vi "Add Namer with Shared Approval File.vi"   [LabVIEW 2020, in "Approval Tests.lvlib"]
doc: "Drops everything needed to have several approval tests share the same approval file."
uses:
  Approval Tests.lvlib
  Options/Options.lvclass
  Namer With Shared Approved File/Namer With Shared Approved File.lvclass
  Namer With Shared Approved File/Namer With Shared Approved File.lvclass/Namer With Shared Approved File.ctl
  Namer With Shared Approved File/Write Shared Approved File Path.vi
  Options/Write Namer.vi
  C:/Users/SAS/Desktop/ApprovalTests.LabVIEW/Source/Approval Tests/Namer/Namer.lvclass
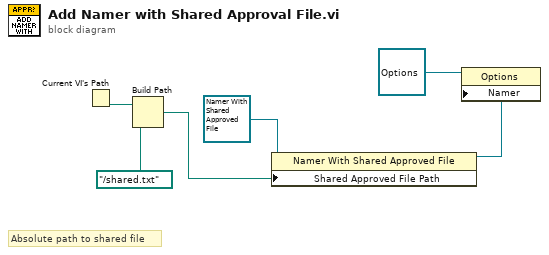
[diagram p0: block diagram]
diagram:
  # "Absolute path to shared file"
  n1 = Current VI's Path() -> (path=w3:path)
  n2 = Build Path(base path=w3, name or relative path=path "../shared.txt" ("Path")) -> (appended path=w1:path)
  n3 = property class="Namer With Shared Approved File"(reference=refnum<class "Namer With Shared Approved File.lvclass"> refnum ("Approval Tests.lvlib:Regex Scrubber"), "Shared Approved File Path"=w1) -> (reference out=w4:refnum<class "Namer With Shared Approved File.lvclass">)  [unwired: 1 in, 1 out]
  n4 = property class="Options"(reference=refnum<class "Options.lvclass"> refnum ("Approval Tests.lvlib:Options"), "Namer"=w4) -> ()  [unwired: 1 in, 2 out]
